vi "serial_cycle_thread_single.vi"() -> ()   [LabVIEW 2020]
doc: "该模板用于创建生产者／消费者模式的应用程序，以事件驱动的方式，生成队列中的项。如需通过响应事件实现代码的异步执行，同时不影响用户界面的响应速度，可考虑用该模式替代“用户界面事件处理器”模式。"
uses:
  <vilib>/Instr/_visa.llb/VISA Set IO Buffer Mask.ctl
  <vilib>/Instr/_visa.llb/VISA Flush IO Buffer Mask.ctl
  <vilib>/Instr/_visa.llb/VISA Configure Serial Port (Instr).vi
panel:
  in  "开等待时间（毫秒） 1":u32
  in  "开等待时间（毫秒）3":u32
  in  "开等待时间（毫秒）2":u32
  in  "开等待时间（毫秒）4":u32
  in  "开等待时间5（毫秒）":u32
  in  "开等待时间6（毫秒）":u32
  in  "开等待时间7（毫秒）":u32
  in  "开等待时间8（毫秒）":u32
  in  "关等待(ms)8":u32
  in  "VISA资源名称8":refnum<visa-resource-name>
  out "读取的数据8":string
  out "数据读取时间8":u32
  in  "COM8":bool
  in  "关等待(ms)7":u32
  in  "VISA资源名称7":refnum<visa-resource-name>
  out "读取的数据7":string
  out "数据读取时间7":u32
  in  "COM7":bool
  in  "关等待(ms)6":u32
  in  "VISA资源名称6":refnum<visa-resource-name>
  out "读取的数据6":string
  out "数据读取时间6":u32
  in  "COM6":bool
  in  "关等待(ms)5":u32
  in  "VISA资源名称5":refnum<visa-resource-name>
  out "读取的数据5":string
  out "数据读取时间5":u32
  in  "COM5":bool
  in  "关等待(ms)4":u32
  in  "VISA资源名称4":refnum<visa-resource-name>
  out "读取的数据4":string
  out "数据读取时间4":u32
  in  "COM4":bool
  out "数据读取时间3":u32
  out "读取的数据3":string
  out "数据读取时间1":u32
  out "读取的数据1":string
  out "数据读取时间2":u32
  out "读取的数据2":string
  in  "写入缓冲区":string="~\u00010000@SCNTRG1;\u0003"
  out "标准码词":string
  in  "关等待(ms)2":u32
  in  "VISA资源名称2":refnum<visa-resource-name>
  in  "VISA资源名称3":refnum<visa-resource-name>
  in  "关等待(ms)3":u32
  in  "关等待(ms)1":u32
  in  "VISA资源名称":refnum<visa-resource-name>
  in  "读取标准码词":bool
  in  "COM3":bool
  in  "COM2":bool
  in  "开始测试":bool
  in  "COM1":bool
  in  "继电器调试":bool
  in  "打开开关":bool
  in  "串口资源":refnum<visa-resource-name>
  in  "stop":bool caption="停止"
  out "错误输出":errorcluster
  out "error out":errorcluster caption="继电器板错误输入输出"
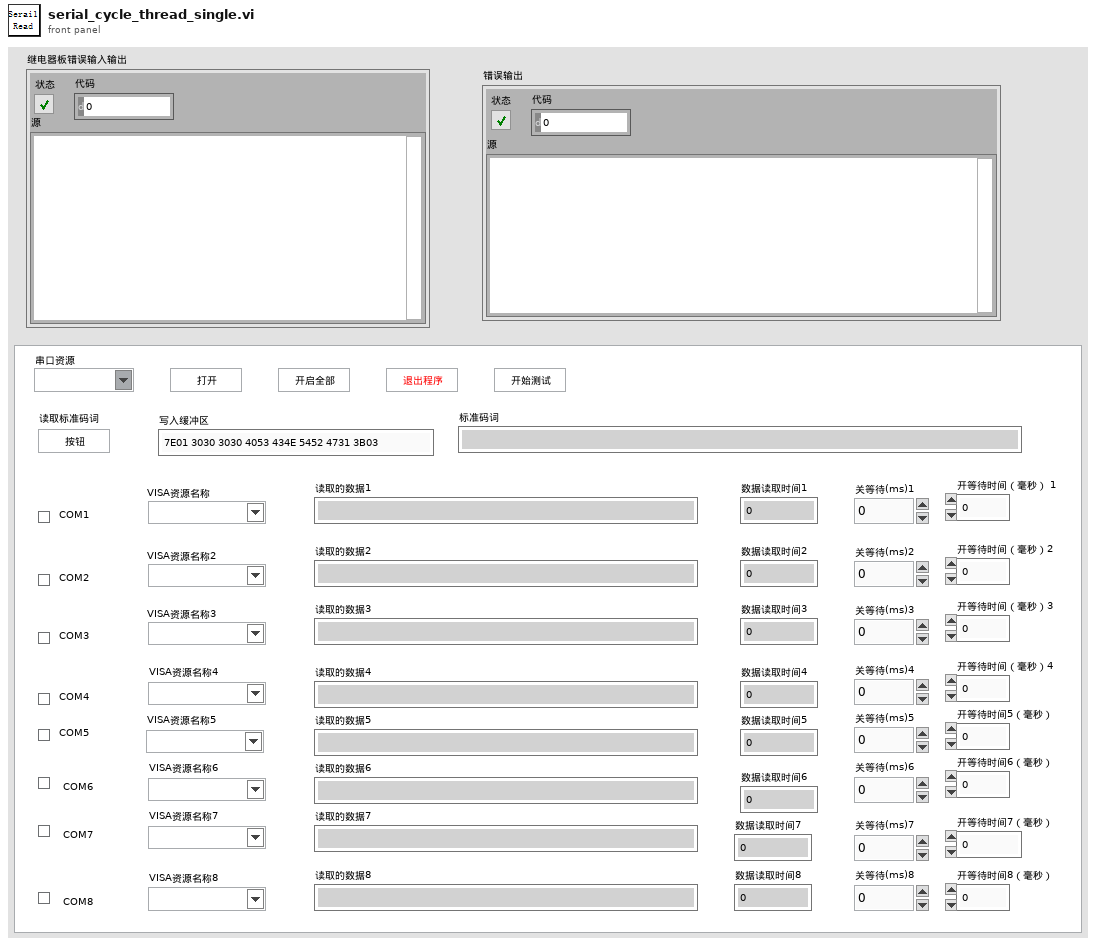
[diagram p1: front panel]
types:
  T1 = typedef "VISA Flush IO Buffer Mask.ctl" = u16
  T2 = typedef "VISA Set IO Buffer Mask.ctl" = u16
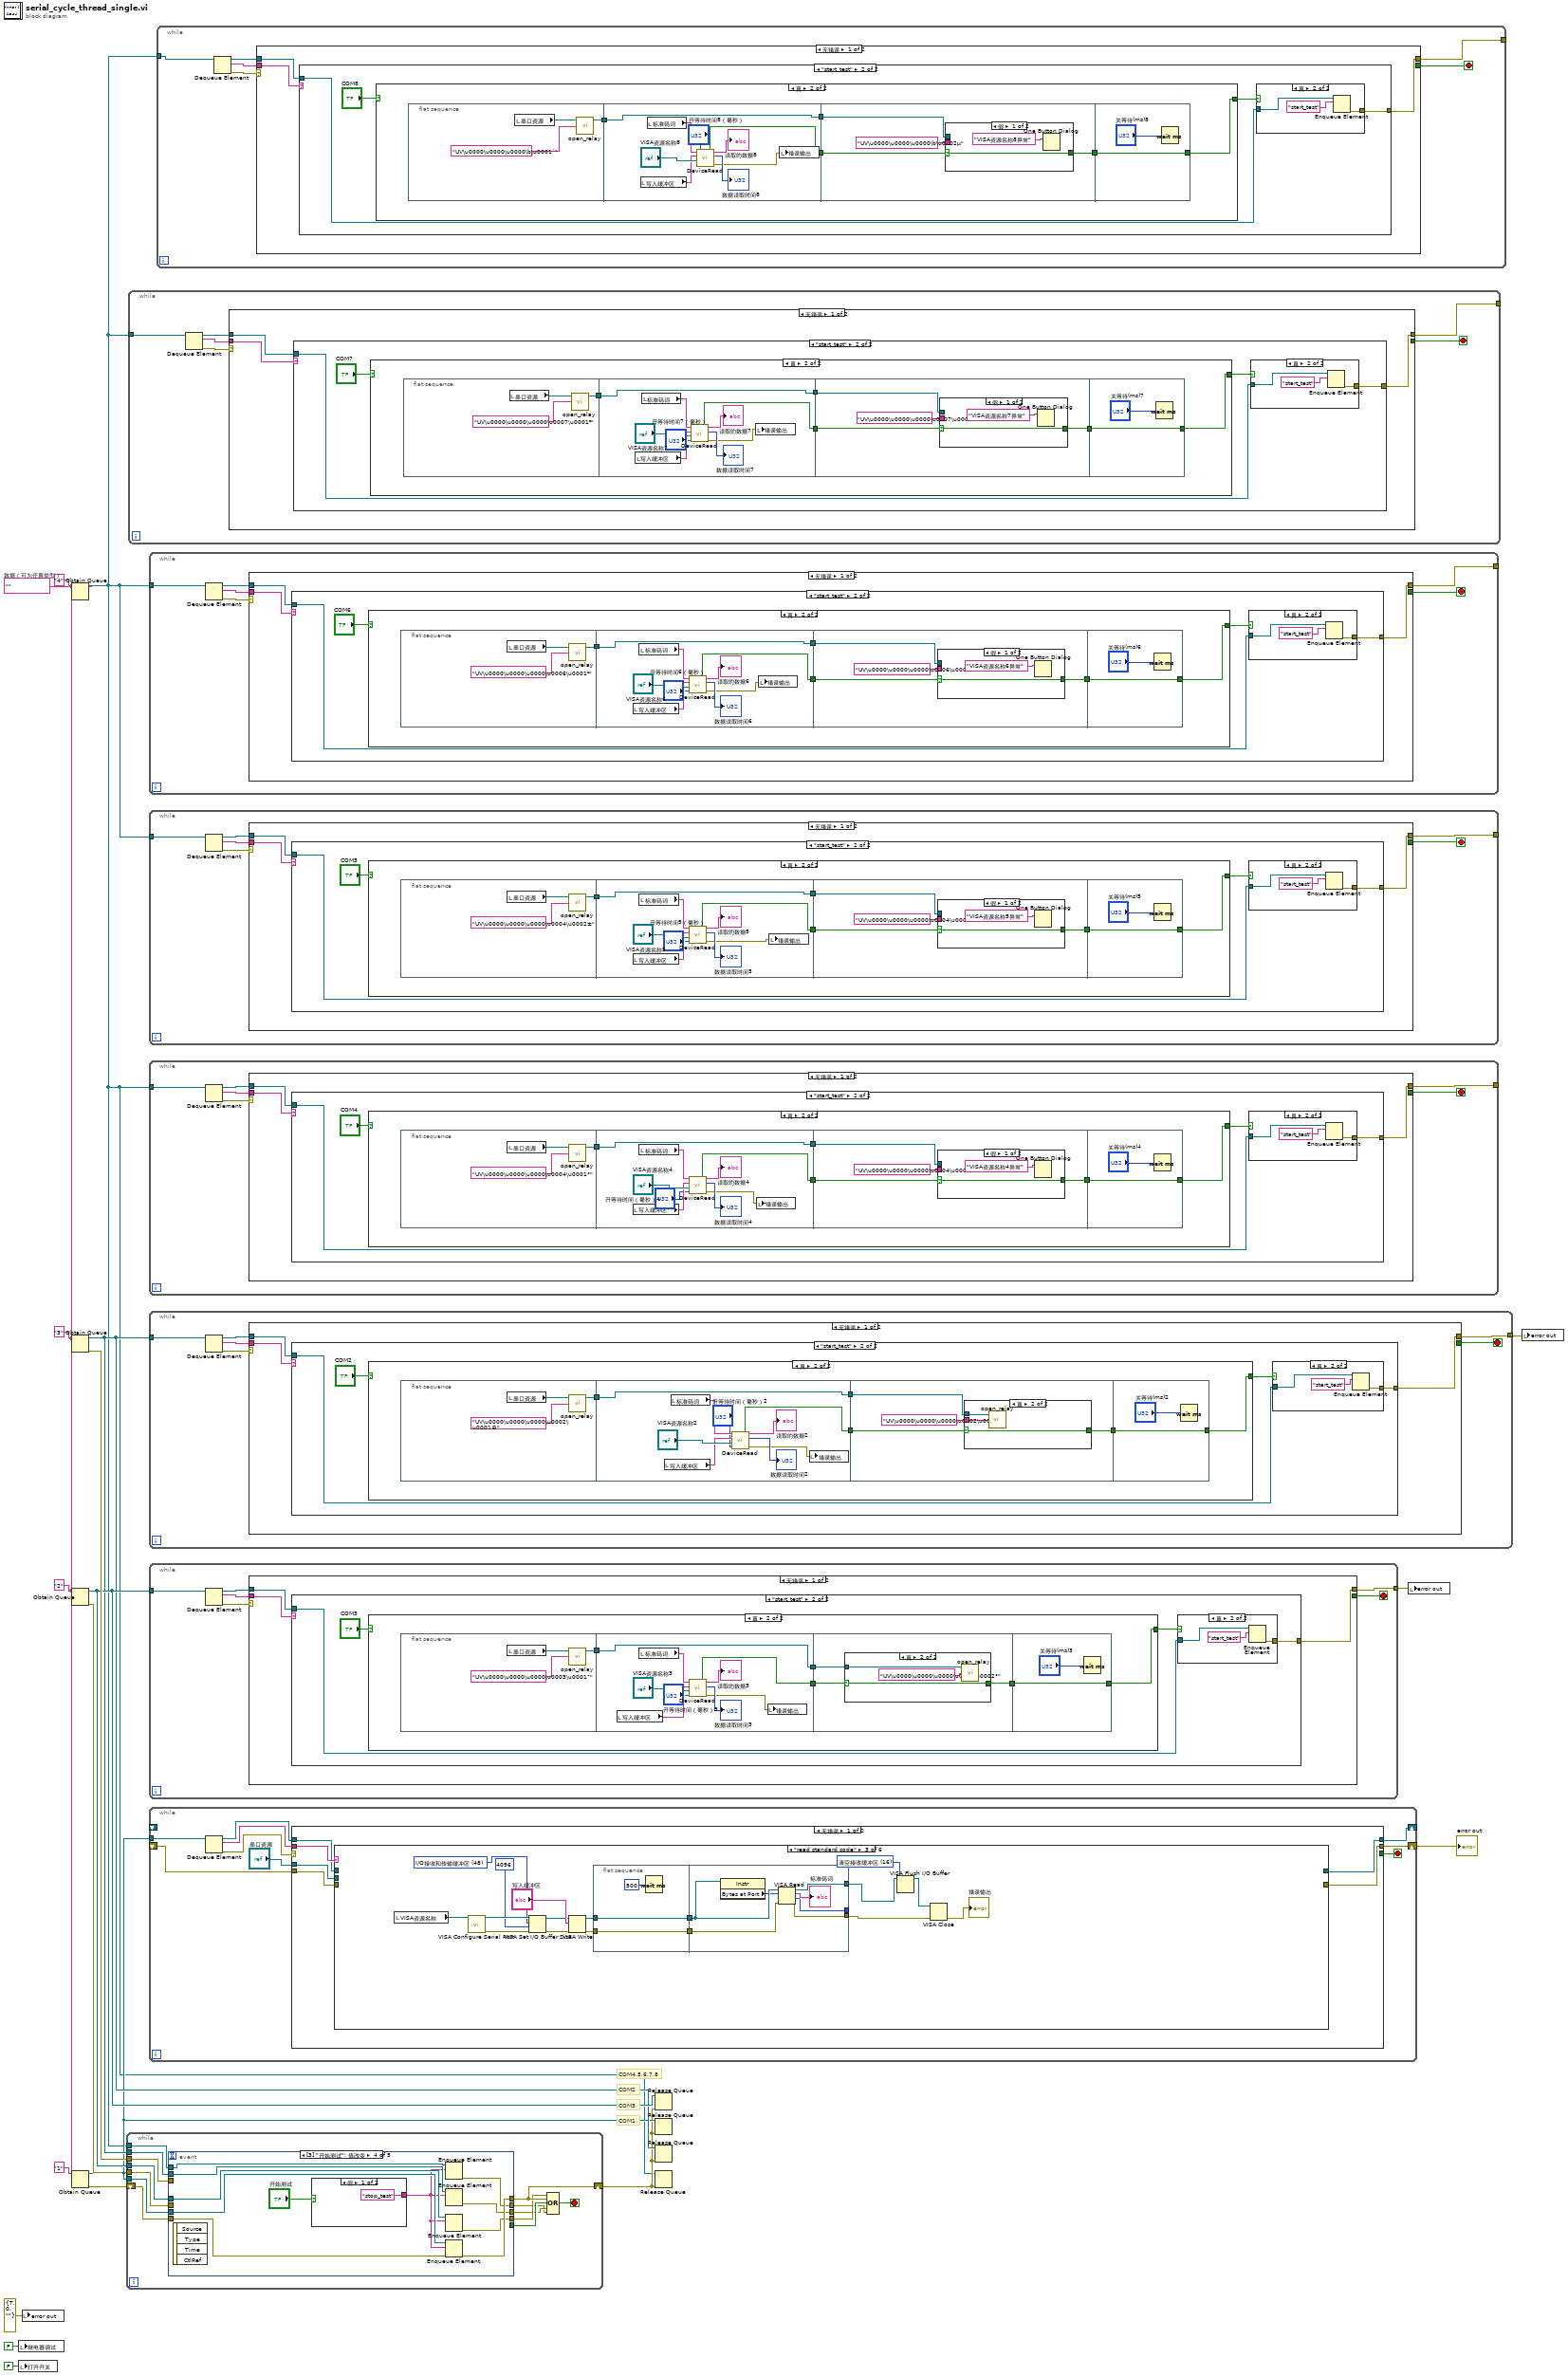
[diagram p0: block diagram]
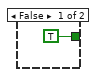
[diagram p4: hidden frame]
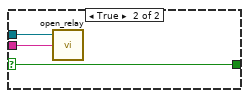
[diagram p5: hidden frame]
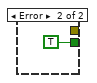
[diagram p6: hidden frame]
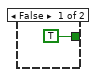
[diagram p9: hidden frame]
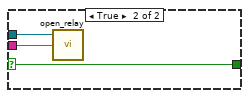
[diagram p10: hidden frame]
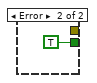
[diagram p11: hidden frame]
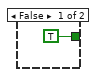
[diagram p14: hidden frame]
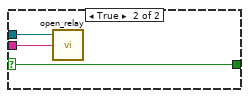
[diagram p15: hidden frame]
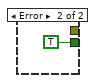
[diagram p16: hidden frame]
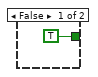
[diagram p19: hidden frame]
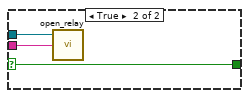
[diagram p20: hidden frame]
diagram:
  w4 = ""  # 数据（可为任意类型）
  # "COM4,5,6,7,8"
  # "COM1"
  # "COM3"
  # "COM2"
  n1 = local write "继电器调试"(FALSE ("继电器调试")) -> ()
  n2 = local write "打开开关"(FALSE ("打开开关")) -> ()
  n3 = local write "error out"(errorcluster {"status"=TRUE, "code"=0, "source"=""} ("error out")) -> ()
  n4 = Obtain Queue(name (unnamed)="4" ("名称（未命名）"), element data type=w4) -> (queue out=w1:refnum<queue>)  [unwired: 3 in, 2 out]
  n5 = Obtain Queue(name (unnamed)="3" ("名称（未命名）"), element data type=w4) -> (queue out=w6:refnum<queue>, error out=w15:errorcluster)  [unwired: 3 in, 1 out]
  n6 = Obtain Queue(name (unnamed)="2" ("名称（未命名）"), element data type=w4) -> (queue out=w10:refnum<queue>, error out=w14:errorcluster)  [unwired: 3 in, 1 out]
  n7 = Obtain Queue(name (unnamed)="1" ("名称（未命名）"), element data type=w4) -> (queue out=w5:refnum<queue>, error out=w19:errorcluster)  [unwired: 3 in, 1 out]
  n8 = while {
    shift-right: [w29] -> w3
    shift-left: w19 -> [w31]
    tunnel: w5 -> [w32]
    tunnel: w15 -> [w26]
    tunnel: w14 -> [w24]
    tunnel: w6 -> [w23]
    tunnel: w10 -> [w22]
    tunnel: w1 -> [w20]
    stop <- w28 stop-if-true
    n9 = event shown="[3] \"开始测试\": 值改变" {
      selector: _ -> [_ _ _ _ _]
      dyn-events: _ -> [_ _ _ _ _]
      timeout: _ -> [_ _ _ _ _]
      tunnel: w32 -> [w37 w42 w48 w58 _]
      tunnel: w31 -> [w36 _ _ w55 w64]
      tunnel: [w35 w43 w47 w59 w64] -> w29
      tunnel: [_ _ _ _ "stop"] -> w30
      tunnel: [_ _ _ w52 w63] -> w27
      tunnel: w26 -> [_ _ _ _ w63]
      tunnel: [_ _ _ w53 w62] -> w25
      tunnel: w24 -> [_ _ _ _ w62]
      tunnel: w23 -> [_ _ _ w56 _]
      tunnel: w22 -> [_ _ _ w54 _]
      tunnel: [_ _ _ w50 _] -> w21
      tunnel: w20 -> [_ _ _ w49 _]
      event "打开开关": Value Change {
        n10 = event-data() -> ()  [unwired: 1 in, 1 out]
        n11 = case shown="假" "打开开关" {
          tunnel: ["close visa" ("element") "open visa" ("element")] -> w33
          frame False {
          }
          frame True {
          }
        }
        n12 = Enqueue Element(queue=w37, element=w33, error in (no error)=w36) -> (error out=w35:errorcluster)  [unwired: 1 in, 2 out]
      }
      event "继电器调试": Value Change {
        n13 = event-data() -> ()  [unwired: 1 in, 3 out]
        n14 = case shown="假" "继电器调试" {
          tunnel: ["close_test" ("元素") "open_test" ("元素")] -> w40
          frame False {
          }
          frame True {
          }
        }
        n15 = Enqueue Element(queue=w42, element=w40) -> (error out=w43:errorcluster)  [unwired: 2 in, 2 out]
      }
      event "读取标准码词": Value Change {
        n16 = event-data() -> ()  [unwired: 1 in, 4 out]
        n17 = Enqueue Element(queue=w48, element="read standard code" ("元素")) -> (error out=w47:errorcluster)  [unwired: 2 in, 2 out]
      }
      event "开始测试": Value Change {
        n18 = event-data() -> ()  [unwired: 1 in, 4 out]
        n19 = case shown="假" "开始测试" {
          tunnel: ["stop_test" ("元素") "start_test" ("元素")] -> w51
          frame False {
          }
          frame True {
          }
        }
        n20 = Enqueue Element(queue=w58, element=w51, error in (no error)=w55) -> (error out=w59:errorcluster)  [unwired: 1 in, 2 out]
        n21 = Enqueue Element(queue=w49, element=w51) -> (error out=w50:errorcluster)  [unwired: 2 in, 2 out]
        n22 = Enqueue Element(queue=w56, element=w51) -> (error out=w53:errorcluster)  [unwired: 2 in, 2 out]
        n23 = Enqueue Element(queue=w54, element=w51) -> (error out=w52:errorcluster)  [unwired: 2 in, 2 out]
      }
      event "stop": Value Change {
        n24 = event-data() -> ()  [unwired: 1 in, 1 out]
      }
    }
    n25 = Compound Arithmetic op=OR ("复合运算")(w27, w29, w30, w25, w21) -> (w28:bool)
  }
  n26 = while {
    tunnel: [w68] -> _
    tunnel: w1 -> [w66]
    stop <- w69 stop-if-true
    n27 = Dequeue Element(queue=w66) -> (queue out=w67:refnum<queue>, element=w70:string, error out=w71:errorcluster)  [unwired: 2 in, 1 out]
    n28 = case shown="无错误" w71 {
      tunnel: w70 -> [w74 _]
      tunnel: [_ TRUE] -> w69
      tunnel: [w73 _] -> w68
      tunnel: w67 -> [w72 _]
      frame No Error {
        n29 = case shown="\"start_test\"" w74 {
          tunnel: [_ w76] -> w73
          tunnel: w72 -> [_ w75]
          frame "假", Default {
          }
          frame "start_test" {
            n30 = case shown="真" "COM7" {
              tunnel: [TRUE w86] -> w77
              frame False {
              }
              frame True {
                n31 = flat-sequence {
                  tunnel: [w89] -> w87
                  tunnel: w87 -> [w93]
                  tunnel: [w96] -> w84
                  tunnel: [w93] -> w83
                  tunnel: [w102] -> w85
                  tunnel: w84 -> [w101]
                  tunnel: w83 -> [w100]
                  tunnel: [w109] -> w86
                  tunnel: w85 -> [w109]
                  frame #0 {
                    n32 = local read "串口资源"() -> (w88:refnum<visa-resource-name>)
                    n33 = call "open_relay.vi"("写入缓冲区"="UV\u0000\u0000\u0000\u0007\u0001³", "VISA资源名称"=w88) -> ("VISA资源名称输出"=w89:refnum<visa-resource-name>)  [unwired: 1 in, 2 out]
                  }
                  frame #1 {
                    n34 = local read "写入缓冲区"() -> (w97:string)
                    n35 = local read "标准码词"() -> (w98:string)
                    n36 = call "DeviceRead.vi"("等待时间（毫秒）"="开等待时间7（毫秒）", "VISA resource name"="VISA资源名称7", "写入缓冲区"=w97, "标准码词"=w98) -> ("错误输出"=w91:errorcluster, "x = y?"=w96:bool, "数据读取时间"=→"数据读取时间7":u32, "连接的字符串"=→"读取的数据7":string)
                    n37 = local write "错误输出"(w91) -> ()
                  }
                  frame #2 {
                    n38 = case shown="假" w101 {
                      selector: w101 -> [w105 w107]
                      tunnel: "UV\u0000\u0000\u0000\u0007\u0002´" ("写入缓冲区") -> [_ w108]
                      tunnel: [w105 w107] -> w102
                      tunnel: w100 -> [_ w106]
                      frame False {
                        n39 = One Button Dialog(message="VISA资源名称7异常" ("消息")) -> ()  [unwired: 1 in, 1 out]
                      }
                      frame True {
                        n40 = call "open_relay.vi"("写入缓冲区"=w108, "VISA资源名称"=w106) -> ()  [unwired: 1 in, 3 out]
                      }
                    }
                  }
                  frame #3 {
                    n41 = Wait (ms)(milliseconds to wait="关等待(ms)7") -> ()  [unwired: 1 out]
                  }
                }
              }
            }
            n42 = case shown="真" w77 {
              tunnel: [_ w80] -> w76
              tunnel: w75 -> [_ w79]
              frame False {
              }
              frame True {
                n43 = Enqueue Element(queue=w79, element="start_test" ("元素")) -> (error out=w80:errorcluster)  [unwired: 2 in, 2 out]
              }
            }
          }
        }
      }
      frame Error {
      }
    }
  }
  n44 = while {
    tunnel: [w114] -> _
    tunnel: w1 -> [w112]
    stop <- w115 stop-if-true
    n45 = Dequeue Element(queue=w112) -> (queue out=w113:refnum<queue>, element=w116:string, error out=w117:errorcluster)  [unwired: 2 in, 1 out]
    n46 = case shown="无错误" w117 {
      tunnel: w116 -> [w120 _]
      tunnel: [_ TRUE] -> w115
      tunnel: [w119 _] -> w114
      tunnel: w113 -> [w118 _]
      frame No Error {
        n47 = case shown="\"start_test\"" w120 {
          tunnel: [_ w122] -> w119
          tunnel: w118 -> [_ w121]
          frame "假", Default {
          }
          frame "start_test" {
            n48 = case shown="真" "COM6" {
              tunnel: [TRUE w132] -> w123
              frame False {
              }
              frame True {
                n49 = flat-sequence {
                  tunnel: [w135] -> w133
                  tunnel: w133 -> [w139]
                  tunnel: [w142] -> w130
                  tunnel: [w139] -> w129
                  tunnel: [w148] -> w131
                  tunnel: w130 -> [w147]
                  tunnel: w129 -> [w146]
                  tunnel: [w155] -> w132
                  tunnel: w131 -> [w155]
                  frame #0 {
                    n50 = local read "串口资源"() -> (w134:refnum<visa-resource-name>)
                    n51 = call "open_relay.vi"("写入缓冲区"="UV\u0000\u0000\u0000\u0006\u0001²", "VISA资源名称"=w134) -> ("VISA资源名称输出"=w135:refnum<visa-resource-name>)  [unwired: 1 in, 2 out]
                  }
                  frame #1 {
                    n52 = local read "写入缓冲区"() -> (w143:string)
                    n53 = local read "标准码词"() -> (w144:string)
                    n54 = call "DeviceRead.vi"("等待时间（毫秒）"="开等待时间6（毫秒）", "VISA resource name"="VISA资源名称6", "写入缓冲区"=w143, "标准码词"=w144) -> ("错误输出"=w137:errorcluster, "x = y?"=w142:bool, "数据读取时间"=→"数据读取时间6":u32, "连接的字符串"=→"读取的数据6":string)
                    n55 = local write "错误输出"(w137) -> ()
                  }
                  frame #2 {
                    n56 = case shown="假" w147 {
                      selector: w147 -> [w151 w153]
                      tunnel: "UV\u0000\u0000\u0000\u0006\u0002³" ("写入缓冲区") -> [_ w154]
                      tunnel: [w151 w153] -> w148
                      tunnel: w146 -> [_ w152]
                      frame False {
                        n57 = One Button Dialog(message="VISA资源名称6异常" ("消息")) -> ()  [unwired: 1 in, 1 out]
                      }
                      frame True {
                        n58 = call "open_relay.vi"("写入缓冲区"=w154, "VISA资源名称"=w152) -> ()  [unwired: 1 in, 3 out]
                      }
                    }
                  }
                  frame #3 {
                    n59 = Wait (ms)(milliseconds to wait="关等待(ms)6") -> ()  [unwired: 1 out]
                  }
                }
              }
            }
            n60 = case shown="真" w123 {
              tunnel: [_ w126] -> w122
              tunnel: w121 -> [_ w125]
              frame False {
              }
              frame True {
                n61 = Enqueue Element(queue=w125, element="start_test" ("元素")) -> (error out=w126:errorcluster)  [unwired: 2 in, 2 out]
              }
            }
          }
        }
      }
      frame Error {
      }
    }
  }
  n62 = while {
    tunnel: [w160] -> _
    tunnel: w1 -> [w158]
    stop <- w161 stop-if-true
    n63 = Dequeue Element(queue=w158) -> (queue out=w159:refnum<queue>, element=w162:string, error out=w163:errorcluster)  [unwired: 2 in, 1 out]
    n64 = case shown="无错误" w163 {
      tunnel: w162 -> [w166 _]
      tunnel: [_ TRUE] -> w161
      tunnel: [w165 _] -> w160
      tunnel: w159 -> [w164 _]
      frame No Error {
        n65 = case shown="\"start_test\"" w166 {
          tunnel: [_ w168] -> w165
          tunnel: w164 -> [_ w167]
          frame "假", Default {
          }
          frame "start_test" {
            n66 = case shown="真" "COM5" {
              tunnel: [TRUE w178] -> w169
              frame False {
              }
              frame True {
                n67 = flat-sequence {
                  tunnel: [w181] -> w179
                  tunnel: w179 -> [w185]
                  tunnel: [w188] -> w176
                  tunnel: [w185] -> w175
                  tunnel: [w194] -> w177
                  tunnel: w176 -> [w193]
                  tunnel: w175 -> [w192]
                  tunnel: [w201] -> w178
                  tunnel: w177 -> [w201]
                  frame #0 {
                    n68 = local read "串口资源"() -> (w180:refnum<visa-resource-name>)
                    n69 = call "open_relay.vi"("写入缓冲区"="UV\u0000\u0000\u0000\u0004\u0002±", "VISA资源名称"=w180) -> ("VISA资源名称输出"=w181:refnum<visa-resource-name>)  [unwired: 1 in, 2 out]
                  }
                  frame #1 {
                    n70 = local read "写入缓冲区"() -> (w189:string)
                    n71 = local read "标准码词"() -> (w190:string)
                    n72 = call "DeviceRead.vi"("等待时间（毫秒）"="开等待时间5（毫秒）", "VISA resource name"="VISA资源名称5", "写入缓冲区"=w189, "标准码词"=w190) -> ("错误输出"=w183:errorcluster, "x = y?"=w188:bool, "数据读取时间"=→"数据读取时间5":u32, "连接的字符串"=→"读取的数据5":string)
                    n73 = local write "错误输出"(w183) -> ()
                  }
                  frame #2 {
                    n74 = case shown="假" w193 {
                      selector: w193 -> [w197 w199]
                      tunnel: "UV\u0000\u0000\u0000\u0004\u0002±" ("写入缓冲区") -> [_ w200]
                      tunnel: [w197 w199] -> w194
                      tunnel: w192 -> [_ w198]
                      frame False {
                        n75 = One Button Dialog(message="VISA资源名称5异常" ("消息")) -> ()  [unwired: 1 in, 1 out]
                      }
                      frame True {
                        n76 = call "open_relay.vi"("写入缓冲区"=w200, "VISA资源名称"=w198) -> ()  [unwired: 1 in, 3 out]
                      }
                    }
                  }
                  frame #3 {
                    n77 = Wait (ms)(milliseconds to wait="关等待(ms)5") -> ()  [unwired: 1 out]
                  }
                }
              }
            }
            n78 = case shown="真" w169 {
              tunnel: [_ w172] -> w168
              tunnel: w167 -> [_ w171]
              frame False {
              }
              frame True {
                n79 = Enqueue Element(queue=w171, element="start_test" ("元素")) -> (error out=w172:errorcluster)  [unwired: 2 in, 2 out]
              }
            }
          }
        }
      }
      frame Error {
      }
    }
  }
  n80 = while {
    tunnel: [w206] -> _
    tunnel: w1 -> [w204]
    stop <- w207 stop-if-true
    n81 = Dequeue Element(queue=w204) -> (queue out=w205:refnum<queue>, element=w208:string, error out=w209:errorcluster)  [unwired: 2 in, 1 out]
    n82 = case shown="无错误" w209 {
      tunnel: w208 -> [w212 _]
      tunnel: [_ TRUE] -> w207
      tunnel: [w211 _] -> w206
      tunnel: w205 -> [w210 _]
      frame No Error {
        n83 = case shown="\"start_test\"" w212 {
          tunnel: [_ w214] -> w211
          tunnel: w210 -> [_ w213]
          frame "假", Default {
          }
          frame "start_test" {
            n84 = case shown="真" "COM4" {
              tunnel: [TRUE w224] -> w215
              frame False {
              }
              frame True {
                n85 = flat-sequence {
                  tunnel: [w227] -> w225
                  tunnel: w225 -> [w231]
                  tunnel: [w234] -> w222
                  tunnel: [w231] -> w221
                  tunnel: [w240] -> w223
                  tunnel: w222 -> [w239]
                  tunnel: w221 -> [w238]
                  tunnel: [w247] -> w224
                  tunnel: w223 -> [w247]
                  frame #0 {
                    n86 = local read "串口资源"() -> (w226:refnum<visa-resource-name>)
                    n87 = call "open_relay.vi"("写入缓冲区"="UV\u0000\u0000\u0000\u0004\u0001°", "VISA资源名称"=w226) -> ("VISA资源名称输出"=w227:refnum<visa-resource-name>)  [unwired: 1 in, 2 out]
                  }
                  frame #1 {
                    n88 = local read "写入缓冲区"() -> (w235:string)
                    n89 = local read "标准码词"() -> (w236:string)
                    n90 = call "DeviceRead.vi"("等待时间（毫秒）"="开等待时间（毫秒）4", "VISA resource name"="VISA资源名称4", "写入缓冲区"=w235, "标准码词"=w236) -> ("错误输出"=w229:errorcluster, "x = y?"=w234:bool, "数据读取时间"=→"数据读取时间4":u32, "连接的字符串"=→"读取的数据4":string)
                    n91 = local write "错误输出"(w229) -> ()
                  }
                  frame #2 {
                    n92 = case shown="假" w239 {
                      selector: w239 -> [w243 w245]
                      tunnel: "UV\u0000\u0000\u0000\u0004\u0002±" ("写入缓冲区") -> [_ w246]
                      tunnel: [w243 w245] -> w240
                      tunnel: w238 -> [_ w244]
                      frame False {
                        n93 = One Button Dialog(message="VISA资源名称4异常" ("消息")) -> ()  [unwired: 1 in, 1 out]
                      }
                      frame True {
                        n94 = call "open_relay.vi"("写入缓冲区"=w246, "VISA资源名称"=w244) -> ()  [unwired: 1 in, 3 out]
                      }
                    }
                  }
                  frame #3 {
                    n95 = Wait (ms)(milliseconds to wait="关等待(ms)4") -> ()  [unwired: 1 out]
                  }
                }
              }
            }
            n96 = case shown="真" w215 {
              tunnel: [_ w218] -> w214
              tunnel: w213 -> [_ w217]
              frame False {
              }
              frame True {
                n97 = Enqueue Element(queue=w217, element="start_test" ("元素")) -> (error out=w218:errorcluster)  [unwired: 2 in, 2 out]
              }
            }
          }
        }
      }
      frame Error {
      }
    }
  }
  n98 = while {
    tunnel: w6 -> [w252]
    tunnel: [w251] -> w8
    stop <- w253 stop-if-true
    n99 = Dequeue Element(queue=w252) -> (queue out=w250:refnum<queue>, element=w254:string, error out=w255:errorcluster)  [unwired: 2 in, 1 out]
    n100 = case shown="无错误" w255 {
      tunnel: w254 -> [w258 _]
      tunnel: [_ TRUE] -> w253
      tunnel: [w257 _] -> w251
      tunnel: w250 -> [w256 _]
      frame No Error {
        n101 = case shown="\"start_test\"" w258 {
          tunnel: [_ w260] -> w257
          tunnel: w256 -> [_ w259]
          frame "假", Default {
          }
          frame "start_test" {
            n102 = case shown="真" "COM2" {
              tunnel: [TRUE w270] -> w261
              frame False {
              }
              frame True {
                n103 = flat-sequence {
                  tunnel: [w273] -> w271
                  tunnel: w271 -> [w277]
                  tunnel: [w280] -> w268
                  tunnel: [w277] -> w267
                  tunnel: [w286] -> w269
                  tunnel: w268 -> [w285]
                  tunnel: w267 -> [w284]
                  tunnel: [w293] -> w270
                  tunnel: w269 -> [w293]
                  frame #0 {
                    n104 = local read "串口资源"() -> (w272:refnum<visa-resource-name>)
                    n105 = call "open_relay.vi"("写入缓冲区"="UV\u0000\u0000\u0000\u0002\u0001®", "VISA资源名称"=w272) -> ("VISA资源名称输出"=w273:refnum<visa-resource-name>)  [unwired: 1 in, 2 out]
                  }
                  frame #1 {
                    n106 = local read "写入缓冲区"() -> (w281:string)
                    n107 = local read "标准码词"() -> (w282:string)
                    n108 = call "DeviceRead.vi"("等待时间（毫秒）"="开等待时间（毫秒）2", "VISA resource name"="VISA资源名称2", "写入缓冲区"=w281, "标准码词"=w282) -> ("错误输出"=w275:errorcluster, "x = y?"=w280:bool, "数据读取时间"=→"数据读取时间2":u32, "连接的字符串"=→"读取的数据2":string)
                    n109 = local write "错误输出"(w275) -> ()
                  }
                  frame #2 {
                    n110 = case shown="真" w285 {
                      selector: w285 -> [w289 w291]
                      tunnel: "UV\u0000\u0000\u0000\u0002\u0002¯" ("写入缓冲区") -> [_ w292]
                      tunnel: [w289 w291] -> w286
                      tunnel: w284 -> [_ w290]
                      frame False {
                        n111 = One Button Dialog(message="VISA资源名称2异常" ("消息")) -> ()  [unwired: 1 in, 1 out]
                      }
                      frame True {
                        n112 = call "open_relay.vi"("写入缓冲区"=w292, "VISA资源名称"=w290) -> ()  [unwired: 1 in, 3 out]
                      }
                    }
                  }
                  frame #3 {
                    n113 = Wait (ms)(milliseconds to wait="关等待(ms)2") -> ()  [unwired: 1 out]
                  }
                }
              }
            }
            n114 = case shown="真" w261 {
              tunnel: [_ w264] -> w260
              tunnel: w259 -> [_ w263]
              frame False {
              }
              frame True {
                n115 = Enqueue Element(queue=w263, element="start_test" ("元素")) -> (error out=w264:errorcluster)  [unwired: 2 in, 2 out]
              }
            }
          }
        }
      }
      frame Error {
      }
    }
  }
  n116 = while {
    tunnel: w10 -> [w298]
    tunnel: [w297] -> w9
    stop <- w299 stop-if-true
    n117 = Dequeue Element(queue=w298) -> (queue out=w296:refnum<queue>, element=w300:string, error out=w301:errorcluster)  [unwired: 2 in, 1 out]
    n118 = case shown="无错误" w301 {
      tunnel: w300 -> [w304 _]
      tunnel: [_ TRUE] -> w299
      tunnel: [w303 _] -> w297
      tunnel: w296 -> [w302 _]
      frame No Error {
        n119 = case shown="\"start_test\"" w304 {
          tunnel: [_ w306] -> w303
          tunnel: w302 -> [_ w305]
          frame "假", Default {
          }
          frame "start_test" {
            n120 = case shown="真" "COM3" {
              tunnel: [TRUE w316] -> w307
              frame False {
              }
              frame True {
                n121 = flat-sequence {
                  tunnel: [w319] -> w317
                  tunnel: w317 -> [w323]
                  tunnel: [w324] -> w314
                  tunnel: [w323] -> w313
                  tunnel: [w332] -> w315
                  tunnel: w314 -> [w331]
                  tunnel: w313 -> [w330]
                  tunnel: [w338] -> w316
                  tunnel: w315 -> [w338]
                  frame #0 {
                    n122 = local read "串口资源"() -> (w318:refnum<visa-resource-name>)
                    n123 = call "open_relay.vi"("写入缓冲区"="UV\u0000\u0000\u0000\u0003\u0001¯", "VISA资源名称"=w318) -> ("VISA资源名称输出"=w319:refnum<visa-resource-name>)  [unwired: 1 in, 2 out]
                  }
                  frame #1 {
                    n124 = local read "写入缓冲区"() -> (w328:string)
                    n125 = local read "标准码词"() -> (w327:string)
                    n126 = call "DeviceRead.vi"("等待时间（毫秒）"="开等待时间（毫秒）3", "VISA resource name"="VISA资源名称3", "写入缓冲区"=w328, "标准码词"=w327) -> ("错误输出"=w321:errorcluster, "x = y?"=w324:bool, "数据读取时间"=→"数据读取时间3":u32, "连接的字符串"=→"读取的数据3":string)
                    n127 = local write "错误输出"(w321) -> ()
                  }
                  frame #2 {
                    n128 = case shown="真" w331 {
                      selector: w331 -> [w334 w336]
                      tunnel: [w334 w336] -> w332
                      tunnel: w330 -> [_ w335]
                      frame False {
                        n129 = One Button Dialog(message="VISA资源名称3异常" ("消息")) -> ()  [unwired: 1 in, 1 out]
                      }
                      frame True {
                        n130 = call "open_relay.vi"("写入缓冲区"="UV\u0000\u0000\u0000\u0003\u0002°", "VISA资源名称"=w335) -> ()  [unwired: 1 in, 3 out]
                      }
                    }
                  }
                  frame #3 {
                    n131 = Wait (ms)(milliseconds to wait="关等待(ms)3") -> ()  [unwired: 1 out]
                  }
                }
              }
            }
            n132 = case shown="真" w307 {
              tunnel: [_ w310] -> w306
              tunnel: w305 -> [_ w309]
              frame False {
              }
              frame True {
                n133 = Enqueue Element(queue=w309, element="start_test" ("元素")) -> (error out=w310:errorcluster)  [unwired: 2 in, 2 out]
              }
            }
          }
        }
      }
      frame Error {
      }
    }
  }
  n134 = while {
    tunnel: w5 -> [w349]
    shift-right: [w345] -> _
    shift-left: _ -> [_]
    shift-right: [w344] -> w18
    shift-left: _ -> [w343]
    stop <- w348 stop-if-true
    n135 = Dequeue Element(queue=w349) -> (queue out=w341:refnum<queue>, element=w346:string, error out=w347:errorcluster)  [unwired: 2 in, 1 out]
    n136 = case shown="无错误" w347 {
      tunnel: [_ TRUE] -> w348
      tunnel: w346 -> [w351 _]
      tunnel: [w355 _] -> w345
      tunnel: "串口资源" -> [w354 w448]
      tunnel: [w352 w446] -> w344
      tunnel: w343 -> [w353 w447]
      tunnel: w341 -> [w350 _]
      frame No Error {
        n137 = case shown="\"read standard code\"" w351 {
          tunnel: [_ _ _ w427 w428 w437] -> w355
          tunnel: w354 -> [w358 w362 _ w424 w430 w439]
          tunnel: w353 -> [w357 _ _ w425 w429 w438]
          tunnel: [w356 w359 _ w426 _ w436] -> w352
          tunnel: w350 -> [_ w361 _ _ _ _]
          frame "close visa", Default {
            n138 = VISA Close(VISA resource name=w358, error in (no error)=w357) -> (error out=w356:errorcluster)
          }
          frame "start_test" {
            n139 = case shown="真" "COM1" {
              tunnel: w362 -> [_ w373]
              tunnel: [TRUE w372] -> w360
              frame False {
              }
              frame True {
                n140 = flat-sequence {
                  tunnel: w373 -> [w377]
                  tunnel: [w375] -> w371
                  tunnel: w371 -> [w380]
                  tunnel: [w381] -> w369
                  tunnel: [w380] -> w368
                  tunnel: [w389] -> w370
                  tunnel: w369 -> [w388]
                  tunnel: w368 -> [w387]
                  tunnel: [w395] -> w372
                  tunnel: w370 -> [w395]
                  frame #0 {
                    n141 = Wait (ms)(milliseconds to wait=u32 1000 ("等待时间（毫秒）")) -> ()  [unwired: 1 out]
                    n142 = call "open_relay.vi"("写入缓冲区"="UV\u0000\u0000\u0000\u0001\u0001­", "VISA资源名称"=w377) -> ("VISA资源名称输出"=w375:refnum<visa-resource-name>)  [unwired: 1 in, 2 out]
                  }
                  frame #1 {
                    n143 = local read "写入缓冲区"() -> (w385:string)
                    n144 = local read "标准码词"() -> (w384:string)
                    n145 = call "DeviceRead.vi"("等待时间（毫秒）"="开等待时间（毫秒） 1", "VISA resource name"="VISA资源名称", "写入缓冲区"=w385, "标准码词"=w384) -> ("错误输出"=w378:errorcluster, "x = y?"=w381:bool, "数据读取时间"=→"数据读取时间1":u32, "连接的字符串"=→"读取的数据1":string)
                    n146 = local write "错误输出"(w378) -> ()
                  }
                  frame #2 {
                    n147 = case shown="真" w388 {
                      selector: w388 -> [w391 w393]
                      tunnel: [w391 w393] -> w389
                      tunnel: w387 -> [_ w392]
                      frame False {
                        n148 = One Button Dialog(message="VISA资源名称异常" ("消息")) -> ()  [unwired: 1 in, 1 out]
                      }
                      frame True {
                        n149 = call "open_relay.vi"("写入缓冲区"="UV\u0000\u0000\u0000\u0001\u0002®", "VISA资源名称"=w392) -> ()  [unwired: 1 in, 3 out]
                      }
                    }
                  }
                  frame #3 {
                    n150 = Wait (ms)(milliseconds to wait="关等待(ms)1") -> ()  [unwired: 1 out]
                  }
                }
              }
            }
            n151 = case shown="真" w360 {
              tunnel: w361 -> [_ w365]
              tunnel: [_ w364] -> w359
              frame False {
              }
              frame True {
                n152 = Enqueue Element(queue=w365, element="start_test" ("元素")) -> (error out=w364:errorcluster)  [unwired: 2 in, 2 out]
              }
            }
          }
          frame "read standard code" {
            w399 = T1 16 items=["清空接收缓冲区"=16, "向设备写入传输缓冲区"=32, "清空接收缓冲区（无I/O）"=64, "清空传输缓冲区"=128] ("Mask")
            w403 = T2 48 items=["I/O接收缓冲区"=16, "I/O传输缓冲区"=32, "I/O接收和传输缓冲区"=48] ("Mask")
            n153 = local read "VISA资源名称"() -> (w413:refnum<visa-resource-name>)
            n154 = call-poly "VISA Configure Serial Port"("VISA resource name"=w413) -> ("VISA resource name out"=w407:refnum<visa-resource-name>, "error out"=w405:errorcluster)  [unwired: 13 in]
            n155 = VISA Set I/O Buffer Size(VISA resource name=w407, mask (16)=w403, size (4096)=u32 4096 ("大小(4096)"), error in (no error)=w405) -> (VISA resource name out=w406:refnum<visa-resource-name>, error out=w404:errorcluster)
            n156 = VISA Write(VISA resource name=w406, write buffer="写入缓冲区", error in (no error)=w404) -> (VISA resource name out=w410:refnum<visa-resource-name>, error out=w411:errorcluster)  [unwired: 1 out]
            n157 = flat-sequence {
              tunnel: w410 -> [w415]
              tunnel: w411 -> [w416]
              tunnel: [w416] -> w409
              tunnel: [w415] -> w408
              tunnel: w409 -> [w420]
              tunnel: w408 -> [w423]
              tunnel: [w419] -> w398
              tunnel: [w418] -> _
              tunnel: [w417] -> w401
              frame #0 {
                n158 = Wait (ms)(milliseconds to wait=u32 500 ("等待时间（毫秒）")) -> ()  [unwired: 1 out]
              }
              frame #1 {
                n159 = property class="Instr"(reference=w423) -> ("Bytes at Port"=w422:u32)  [unwired: 1 in, 2 out]
                n160 = VISA Read(VISA resource name=w423, byte count=w422, error in (no error)=w420) -> (VISA resource name out=w419:refnum<visa-resource-name>, read buffer=→"标准码词":string, return count=w418:u32, error out=w417:errorcluster)
              }
            }
            n161 = VISA Flush I/O Buffer(VISA resource name=w398, mask (16)=w399) -> (VISA resource name out=w397:refnum<visa-resource-name>)  [unwired: 1 in, 1 out]
            n162 = VISA Close(VISA resource name=w397, error in (no error)=w401) -> (error out=→"错误输出":errorcluster)
          }
          frame "open visa" {
            n163 = call-poly "VISA Configure Serial Port"("VISA resource name"=w424, "error in (no error)"=w425) -> ("VISA resource name out"=w427:refnum<visa-resource-name>, "error out"=w426:errorcluster)  [unwired: 12 in]
          }
          frame "open_test" {
            n164 = flat-sequence {
              tunnel: w430 -> [w435]
              tunnel: w429 -> [w433]
              tunnel: [w431] -> w428
              frame #0 {
                n165 = Wait (ms)(milliseconds to wait=u32 200 ("等待时间（毫秒）")) -> ()  [unwired: 1 out]
                n166 = VISA Write(VISA resource name=w435, write buffer="UV\u0000\u0000\u0000\u0000\u0007²" ("写入缓冲区"), error in (no error)=w433) -> (VISA resource name out=w431:refnum<visa-resource-name>)  [unwired: 2 out]
              }
            }
          }
          frame "close_test" {
            n167 = flat-sequence {
              tunnel: w439 -> [w444]
              tunnel: w438 -> [w443]
              tunnel: [w441] -> w437
              tunnel: [w440] -> w436
              frame #0 {
                n168 = Wait (ms)(milliseconds to wait=u32 200 ("等待时间（毫秒）")) -> ()  [unwired: 1 out]
                n169 = VISA Write(VISA resource name=w444, write buffer="UV\u0000\u0000\u0000\u0000\b³" ("写入缓冲区"), error in (no error)=w443) -> (VISA resource name out=w441:refnum<visa-resource-name>, error out=w440:errorcluster)  [unwired: 1 out]
              }
            }
          }
        }
      }
      frame Error {
        # "对任意分支返回真，使循环停止运行。"
        n170 = VISA Close(VISA resource name=w448, error in (no error)=w447) -> (error out=w446:errorcluster)
      }
    }
  }
  "error out" <- w18
  n171 = while {
    tunnel: [w452] -> _
    tunnel: w1 -> [w450]
    stop <- w453 stop-if-true
    n172 = Dequeue Element(queue=w450) -> (queue out=w451:refnum<queue>, element=w454:string, error out=w455:errorcluster)  [unwired: 2 in, 1 out]
    n173 = case shown="无错误" w455 {
      tunnel: w454 -> [w458 _]
      tunnel: [_ TRUE] -> w453
      tunnel: [w457 _] -> w452
      tunnel: w451 -> [w456 _]
      frame No Error {
        n174 = case shown="\"start_test\"" w458 {
          tunnel: [_ w460] -> w457
          tunnel: w456 -> [_ w459]
          frame "假", Default {
          }
          frame "start_test" {
            n175 = case shown="真" "COM8" {
              tunnel: [TRUE w470] -> w461
              frame False {
              }
              frame True {
                n176 = flat-sequence {
                  tunnel: [w473] -> w471
                  tunnel: w471 -> [w477]
                  tunnel: [w480] -> w468
                  tunnel: [w477] -> w467
                  tunnel: [w486] -> w469
                  tunnel: w468 -> [w485]
                  tunnel: w467 -> [w484]
                  tunnel: [w493] -> w470
                  tunnel: w469 -> [w493]
                  frame #0 {
                    n177 = local read "串口资源"() -> (w472:refnum<visa-resource-name>)
                    n178 = call "open_relay.vi"("写入缓冲区"="UV\u0000\u0000\u0000\b\u0001´", "VISA资源名称"=w472) -> ("VISA资源名称输出"=w473:refnum<visa-resource-name>)  [unwired: 1 in, 2 out]
                  }
                  frame #1 {
                    n179 = local read "写入缓冲区"() -> (w481:string)
                    n180 = local read "标准码词"() -> (w482:string)
                    n181 = call "DeviceRead.vi"("等待时间（毫秒）"="开等待时间8（毫秒）", "VISA resource name"="VISA资源名称8", "写入缓冲区"=w481, "标准码词"=w482) -> ("错误输出"=w475:errorcluster, "x = y?"=w480:bool, "数据读取时间"=→"数据读取时间8":u32, "连接的字符串"=→"读取的数据8":string)
                    n182 = local write "错误输出"(w475) -> ()
                  }
                  frame #2 {
                    n183 = case shown="假" w485 {
                      selector: w485 -> [w489 w491]
                      tunnel: "UV\u0000\u0000\u0000\b\u0002µ" ("写入缓冲区") -> [_ w492]
                      tunnel: [w489 w491] -> w486
                      tunnel: w484 -> [_ w490]
                      frame False {
                        n184 = One Button Dialog(message="VISA资源名称8异常" ("消息")) -> ()  [unwired: 1 in, 1 out]
                      }
                      frame True {
                        n185 = call "open_relay.vi"("写入缓冲区"=w492, "VISA资源名称"=w490) -> ()  [unwired: 1 in, 3 out]
                      }
                    }
                  }
                  frame #3 {
                    n186 = Wait (ms)(milliseconds to wait="关等待(ms)8") -> ()  [unwired: 1 out]
                  }
                }
              }
            }
            n187 = case shown="真" w461 {
              tunnel: [_ w464] -> w460
              tunnel: w459 -> [_ w463]
              frame False {
              }
              frame True {
                n188 = Enqueue Element(queue=w463, element="start_test" ("元素")) -> (error out=w464:errorcluster)  [unwired: 2 in, 2 out]
              }
            }
          }
        }
      }
      frame Error {
      }
    }
  }
  n189 = Release Queue(queue=w10, error in (no error)=w3) -> ()  [unwired: 1 in, 3 out]
  n190 = Release Queue(queue=w5, error in (no error)=w3) -> ()  [unwired: 1 in, 3 out]
  n191 = Release Queue(queue=w6, error in (no error)=w3) -> ()  [unwired: 1 in, 3 out]
  n192 = Release Queue(queue=w1, error in (no error)=w3) -> ()  [unwired: 1 in, 3 out]
  n193 = local write "error out"(w9) -> ()
  n194 = local write "error out"(w8) -> ()
